vi "Replace_Saved_Coordinates-2.vi"(1 "Index of staring point":i32, 2 "(X,Y,dX,dY) Frame IN":dbl[](array[numeric])) -> (0 "Replaced array":dbl[](array[numeric]))   [LabVIEW 2013]
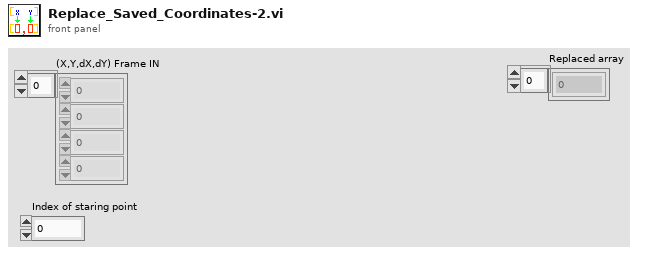
[diagram p1: front panel]
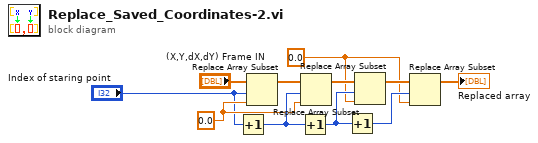
[diagram p0: block diagram]
diagram:
  w4 = 0.0 ("new element/subarray")
  w8 = 0.0 ("new element/subarray")
  n1 = Increment(x="Index of staring point") -> (x+1=w9:i32)
  n2 = Replace Array Subset(array="(X,Y,dX,dY) Frame IN", new element=w8, index="Index of staring point") -> (w11:dbl[])
  n3 = Increment(x=w9) -> (x+1=w7:i32)
  n4 = Replace Array Subset(array=w11, new element=w8, index=w9) -> (w10:dbl[])
  n5 = Increment(x=w7) -> (x+1=w5:i32)
  n6 = Replace Array Subset(array=w10, new element=w4, index=w7) -> (w6:dbl[])
  n7 = Replace Array Subset(array=w6, new element=w4, index=w5) -> (→"Replaced array":dbl[])
